vi "JSONToPackets.vi"(8 "ErrorIn":errorcluster, 11 "JSONIn":refnum<class "JSON Value.lvclass">) -> (0 "ErrorOut":errorcluster, 2 "Packets":T1[](array[typedef]) {"MeasurementConfig"."Resolution[b]" min=4 max=16 step=1; "MeasurementConfig"."Frequency" min=1 max=10000000 step=1}, 3 "JSONOut":refnum<class "JSON Value.lvclass">)   [LabVIEW 2016]
doc: "Convert JSON to Packets"
uses:
  FallSensor/Packet.ctl
  FallSensor/Sample.ctl
  FallSensor/Reading.ctl
  FallSensor/MeasurementConfig.ctl
  FallSensor/Measurement/AccelFSRange.ctl
  FallSensor/Measurement/GyroFSRange.ctl
  <vilib>/addons/JSON API/JSON Value/JSON Value.lvclass
  <vilib>/addons/JSON API/JSON Value/Get Object Item by Name.vi
  <vilib>/addons/JSON API/JSON Array/Get Array.vi
  <vilib>/addons/JSON API/Get Polymorphic/JSON GetSet.lvlib
  <vilib>/addons/JSON API/JSON Array/JSON Array.lvclass
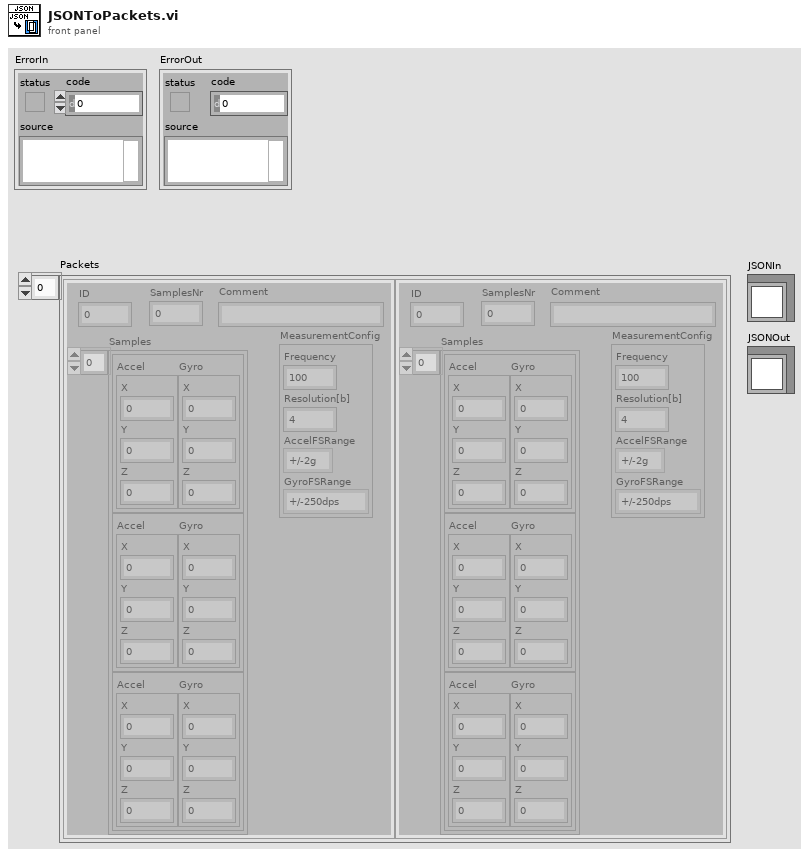
[diagram p1: front panel]
types:
  T1 = typedef "Packet.ctl" = cluster{"ID":u32, "SamplesNr":u32, "Samples":T2[], "MeasurementConfig":T4, "Comment":string}
  T2 = typedef "Sample.ctl" = cluster{"Accel":T3, "Gyro":T3}
  T3 = typedef "Reading.ctl" = cluster{"X":i16, "Y":i16, "Z":i16}
  T4 = typedef "MeasurementConfig.ctl" = cluster{"Frequency":u32, "Resolution[b]":u32, "AccelFSRange":T5, "GyroFSRange":T6}
  T5 = typedef "AccelFSRange.ctl" = enum16{"+/-2g", "+/-4g", "+/-8g", "+/-16g"}
  T6 = typedef "GyroFSRange.ctl" = enum16{"+/-250dps", "+/-500dps", "+/-1000dps", "+/-2000dps"}
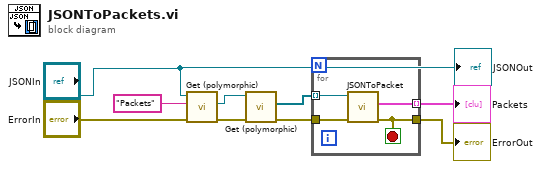
[diagram p0: block diagram]
diagram:
  n1 = call-poly <vilib>:"Get (polymorphic).vi"("error in (no error)"="ErrorIn", "name"="Packets", "JSON Value In"="JSONIn") -> ("error out"=w3:errorcluster, "Value"=w5:refnum<class "JSON Value.lvclass">)  [unwired: 5 in, 2 out]
  n2 = call-poly <vilib>:"Get (polymorphic).vi"("error in (no error)"=w3, "JSON Array in"=w5) -> ("error out"=w4:errorcluster, "Array"=w2:refnum<class "JSON Value.lvclass">[])  [unwired: 7 in, 1 out]
  n3 = for {
    tunnel: [w13] -> w8 mode=indexing
    tunnel: [w12] -> w7
    tunnel: w2 -> [w11] mode=indexing
    tunnel: w4 -> [w10]
    stop <- w12 stop-if-true
    n4 = call "JSONToPacket.vi"("ErrorIn"=w10, "JSONIn"=w11) -> ("ErrorOut"=w12:errorcluster, "Packet"=w13:T1)  [unwired: 7 in, 1 out]
  }
  "ErrorOut" <- w7
  "Packets" <- w8
  "JSONOut" <- "JSONIn"
